vi "LR 700 convert responce.vi"(3 "LR 700 Responce":string) -> (0 "Resistance":dbl format="%.4e")   [LabVIEW 2015]
panel:
  in  "FACTOR":dbl[](array[numeric])=[1e-06, 0.001, 1.0, 1000.0] format="%.0e"
  in  "MULT":string[](array[string])=["U", "M", " ", "K"]
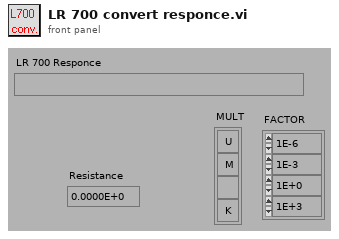
[diagram p1: front panel]
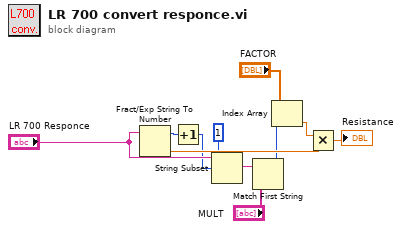
[diagram p0: block diagram]
diagram:
  n1 = Fract/Exp String To Number(string="LR 700 Responce") -> (offset past number=w2:i32, number=w10:dbl)  [unwired: 3 out]
  n2 = Increment(x=w2) -> (x+1=w3:i32)
  n3 = String Subset(string="LR 700 Responce", offset (0)=w3, length (rest)=1) -> (substring=w5:string)
  n4 = Match First String(2:"MULT", 3:w5) -> (0:w9:i32)  [unwired: 1 out]
  n5 = Index Array(array="FACTOR", index=w9) -> (element=w11:dbl)
  n6 = Multiply(x=w11, y=w10) -> (x*y=→"Resistance":dbl)
